vi "10- Push button with event structure.vi"() -> ()   [LabVIEW 2019]
panel:
  in  "?":bool
  out "String":string
  in  "Cluster":cluster{bool, bool, bool, bool, bool}
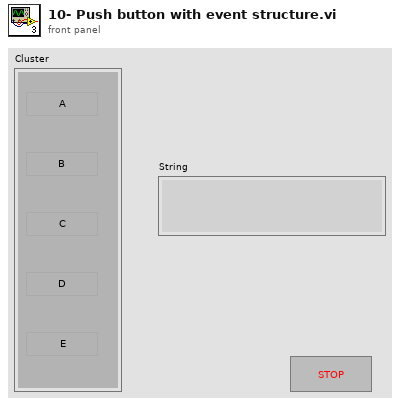
[diagram p1: front panel]
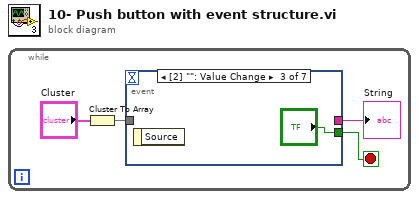
[diagram p0: block diagram]
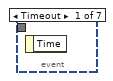
[diagram p2: hidden frame]
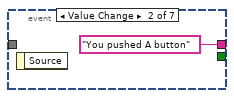
[diagram p3: hidden frame]
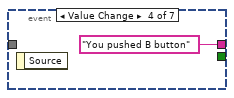
[diagram p4: hidden frame]
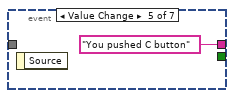
[diagram p5: hidden frame]
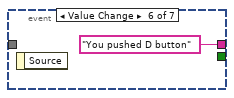
[diagram p6: hidden frame]
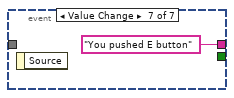
[diagram p7: hidden frame]
diagram:
  n1 = while {
    stop <- w1 stop-if-true
    n2 = Cluster To Array(cluster="Cluster") -> (array=w2:bool[])
    n3 = event shown="[2] \"\": Value Change" {
      selector: _ -> [_ _ _ _ _ _ _]
      dyn-events: _ -> [_ _ _ _ _ _ _]
      timeout: _ -> [_ _ _ _ _ _ _]
      tunnel: [_ "You pushed A button" _ "You pushed B button" "You pushed C button" "You pushed D button" "You pushed E button"] -> w3
      tunnel: w2 -> [_ _ _ _ _ _ _]
      tunnel: [_ _ "?" _ _ _ _] -> w1
      event Timeout {
        n4 = event-data() -> ()  [unwired: 1 in, 1 out]
      }
      event "Cluster.": Value Change {
        n5 = event-data() -> ()  [unwired: 1 in, 1 out]
      }
      event Value Change {
        n6 = event-data() -> ()  [unwired: 1 in, 1 out]
      }
      event "Cluster.": Value Change {
        n7 = event-data() -> ()  [unwired: 1 in, 1 out]
      }
      event "Cluster.": Value Change {
        n8 = event-data() -> ()  [unwired: 1 in, 1 out]
      }
      event "Cluster.": Value Change {
        n9 = event-data() -> ()  [unwired: 1 in, 1 out]
      }
      event "Cluster.": Value Change {
        n10 = event-data() -> ()  [unwired: 1 in, 1 out]
      }
    }
    "String" <- w3
  }
